vi "Launcher.vi"() -> ()   [LabVIEW 2014, in "HIJ 3 Alignment Cams App.lvlib"]
uses:
  HIJ 3 Alignment Cams App.lvlib
  HIJ 3 Aligment Cams Launcher/HIJ 3 Aligment Cams Launcher.lvclass
  HIJ 3 Alignment Cams App/HIJ 3 Alignment Cams App.lvclass
  HIJ Vision Launcher/HIJ Vision Launcher/HIJ Vision Launcher.lvclass/HIJ Vision Launcher.ctl
  <vilib>/ActorFramework/Message Enqueuer/Message Enqueuer.lvclass/Message Enqueuer.ctl
  HIJ Vision Launcher/HIJ Vision Launcher/Write HIJ Vision Camera App.vi
  <vilib>/ActorFramework/Message Enqueuer/Enqueue.vi
  <vilib>/ActorFramework/Message Priority Queue/Priority Enqueue.vi
  Viewable Actor/ViewableActor Messages/Open Front Panel Msg/Open Front Panel Msg.lvclass
  <vilib>/ActorFramework/Actor/Actor.lvclass
panel:
  out "error out":errorcluster
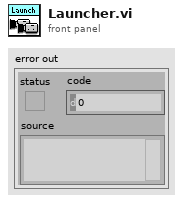
[diagram p1: front panel]
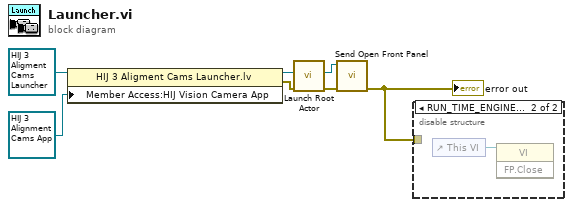
[diagram p0: block diagram]
diagram:
  n1 = property class="HIJ 3 Aligment Cams Launcher.lv"(reference=refnum<class "HIJ 3 Aligment Cams Launcher.lvclass"> refnum ("HIJ 4 Alignment Cams App.lvlib:HIJ 4 Aligment Cams Launcher.lvclass"), "Member Access:HIJ Vision Camera App"=refnum<class "HIJ 3 Alignment Cams App.lvclass"> refnum ("HIJ 4 Alignment Cams App.lvlib:HIJ 4 Alignment Cams App.lvclass")) -> (reference out=w4:refnum<class "HIJ 3 Aligment Cams Launcher.lvclass">, error out=w2:errorcluster)  [unwired: 1 in]
  n2 = call <vilib>:"Launch Root Actor.vi"("error in (no error)"=w2, "Actor"=w4) -> ("error out"=w7:errorcluster, "Actor's Enqueuer"=w6:refnum<class "Message Enqueuer.lvclass">)  [unwired: 8 in]
  n3 = call "Send Open Front Panel.vi"("error in (no error)"=w7, "Message Enqueuer"=w6) -> ("error out"=w1:errorcluster)  [unwired: 8 in, 1 out]
  "error out" <- w1
  n4 = disable-structure shown="RUN_TIME_ENGINE==True" {
    disable-tunnel: w1 -> [_ _]
    frame condition #0 (active) {
    }
    frame condition #1 {
      n5 = control-ref of="This VI"() -> (w8:refnum<vi>)
      n6 = invoke class="VI" method="FP.Close"(reference=w8) -> ()  [unwired: 2 in, 3 out]
    }
  }
